vi "REST API Example - 2.vi"() -> ()   [LabVIEW 2023, in "LabVIEW LLM.lvlib"]
uses:
  LabVIEW LLM.lvlib
  chat-completion non-stream response.ctl
  openai_message.ctl
  chat-completion req.ctl
  <vilib>/httpClient/POSTBuffer.vi
  <vilib>/httpClient/LabVIEWHTTPClient.lvlib
  <vilib>/addons/_JKI.lib/Serialization/JSON/JKI JSON Serialization.lvlib
panel:
  out "应答":T1
  out "error out":errorcluster
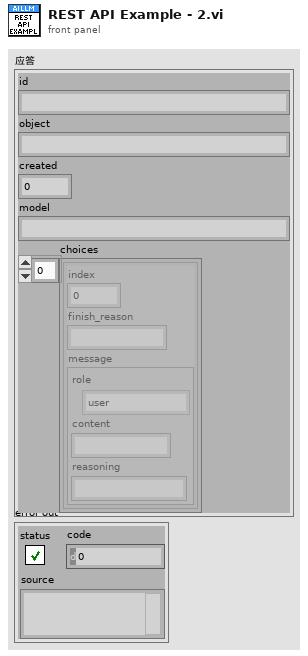
[diagram p1: front panel]
types:
  T1 = typedef "LabVIEW LLM.lvlib/chat-completion non-stream response.ctl" = cluster{"id":string, "object":string, "created":i64, "model":string, "choices":cluster{"index":i64, "finish_reason":string, "message":T2}[]}
  T2 = typedef "LabVIEW LLM.lvlib/openai_message.ctl" = cluster{"role":enum16{"system", "user", "assistant"}, "content":string, "reasoning":string}
  T3 = typedef "LabVIEW LLM.lvlib/chat-completion req.ctl" = cluster{"model":string, "messages":T2[], "max_tokens":u32, "temperature":dbl, "stream":bool, "reasoning":cluster{"effort":enum16{"high", "medium", "low"}, "exclude":bool}}
  T4 = typedef "LabVIEWHTTPClient.lvlib/ClientHandle.ctl" = refnum<k1>
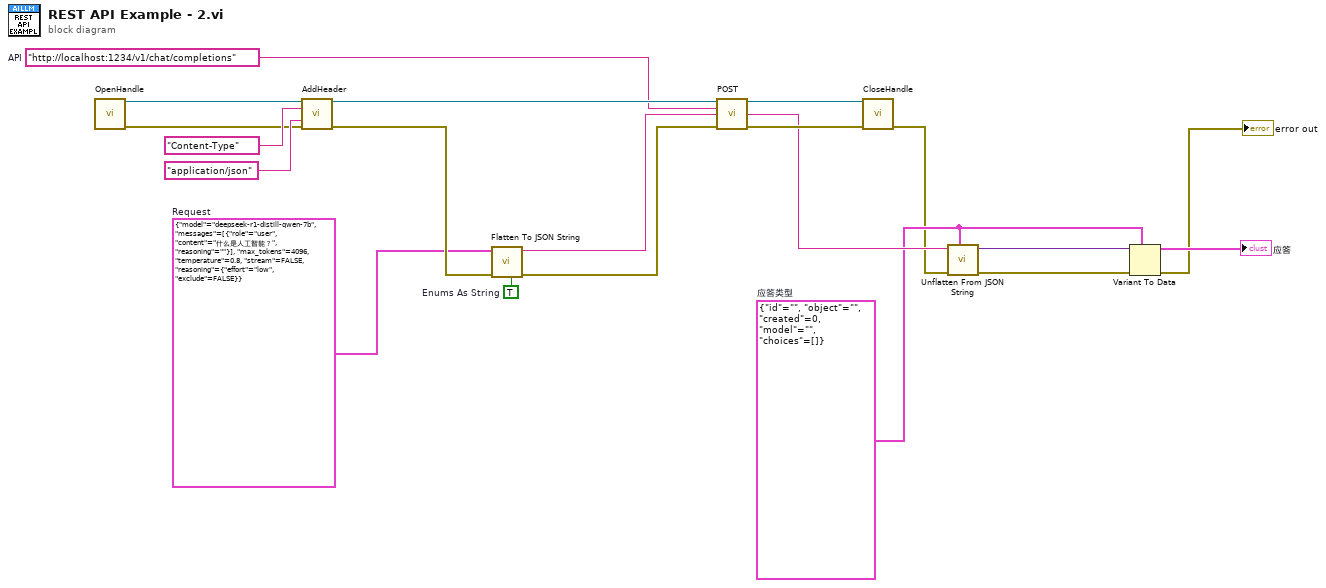
[diagram p0: block diagram]
diagram:
  w4 = T1 {"id"="", "object"="", "created"=0, "model"="", "choices"=[]}  # 应答类型
  w12 = T3 {"model"="deepseek-r1-distill-qwen-7b", "messages"=[{"role"=enum."user", "content"="什么是人工智能？", "reasoning"=""}], "max_tokens"=4096, "temperature"=0.8, "stream"=FALSE, "reasoning"={"effort"=enum."low", "exclude"=FALSE}}  # Request
  w13 = TRUE  # Enums As String
  w14 = "http://localhost:1234/v1/chat/completions"  # API
  n1 = call <vilib>:"OpenHandle.vi"() -> ("client handle out"=w11:T4, "error out"=w10:errorcluster)  [unwired: 14 in]
  n2 = call <vilib>:"AddHeader.vi"("client handle"=w11, "header"="Content-Type", "value"="application/json", "error in (no error)"=w10) -> ("client handle out"=w17:T4, "error out"=w16:errorcluster)  [unwired: 10 in]
  n3 = call <vilib>:"Flatten To JSON String.vi"("Enums As String (F)"=w13, "error in (no error)"=w16, "Variant"=w12) -> ("error out"=w15:errorcluster, "JSON String"=w20:string)  [unwired: 7 in]
  n4 = call-poly <vilib>:"POST.vi"("client handle"=w17, "url"=w14, "buffer"=w20, "error in (no error)"=w15) -> ("client handle out"=w9:T4, "body"=w7:string, "error out"=w8:errorcluster)  [unwired: 8 in, 1 out]
  n5 = call <vilib>:"CloseHandle.vi"("client handle"=w9, "error in (no error)"=w8) -> ("error out"=w2:errorcluster)  [unwired: 13 in]
  n6 = call <vilib>:"Unflatten From JSON String.vi"("Type and Defaults"=w4, "error in (no error)"=w2, "JSON String"=w7) -> ("error out"=w5:errorcluster, "Variant"=w6:variant)  [unwired: 7 in]
  n7 = Variant To Data(error in=w5, type=w4, Variant=w6) -> (data=→"应答":T1, error out=→"error out":errorcluster)
